vi "_tools_protoc.vi"   [LabVIEW 2020]
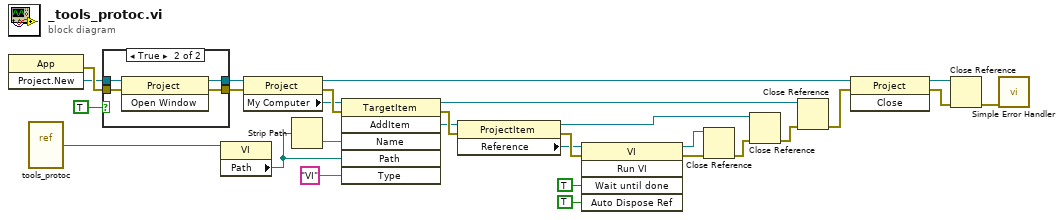
[diagram p0: block diagram]
diagram:
  n1 = invoke class="App" method="Project.New"() -> (error out=w28:errorcluster, "Project:New"=w4:refnum<vi>)  [unwired: 3 in, 1 out]
  n2 = vi-ref "tools_protoc.vi"() -> (w23:refnum<vi>)
  n3 = case shown="True" TRUE {
    tunnel: w4 -> [w30 w34]
    tunnel: w28 -> [w29 w33]
    tunnel: [w30 w32] -> w3
    tunnel: [w29 w31] -> w2
    frame False {
    }
    frame True {
      n4 = invoke class="Project" method="Open Window"(reference=w34, error in=w33) -> (reference out=w32:refnum<vi>, error out=w31:errorcluster)  [unwired: 1 in, 1 out]
    }
  }
  n5 = property class="VI"(reference=w23) -> ("Path"=w22:path)  [unwired: 1 in, 2 out]
  n6 = property class="Project"(reference=w3, error in=w2) -> (reference out=w9:refnum<vi>, error out=w27:errorcluster, "My Computer"=w24:refnum<vi>)
  n7 = Strip Path(path=w22) -> (name=w21:string)  [unwired: 1 out]
  n8 = invoke class="TargetItem" method="AddItem"(reference=w24, error in=w27, "Name"=w21, "Path"=w22, "Type"="VI") -> (reference out=w11:refnum<vi>, error out=w26:errorcluster, "AddItem"=w19:refnum<vi>)  [unwired: 1 in, 3 out]
  n9 = property class="ProjectItem"(reference=w19, error in=w26) -> (reference out=w12:refnum<vi>, error out=w25:errorcluster, "Reference"=w18:refnum<vi>)
  n10 = invoke class="VI" method="Run VI"(reference=w18, error in=w25, "Wait until done"=TRUE ("Wait Until Done"), "Auto Dispose Ref"=TRUE ("Auto Dispose Reference")) -> (reference out=w14:refnum<vi>, error out=w15:errorcluster)  [unwired: 1 in, 3 out]
  n11 = Close Reference(reference=w14, error in (no error)=w15) -> (error out=w13:errorcluster)
  n12 = Close Reference(reference=w12, error in (no error)=w13) -> (error out=w10:errorcluster)
  n13 = Close Reference(reference=w11, error in (no error)=w10) -> (error out=w8:errorcluster)
  n14 = invoke class="Project" method="Close"(reference=w9, error in=w8) -> (reference out=w7:refnum<vi>, error out=w6:errorcluster)  [unwired: 1 in, 1 out]
  n15 = Close Reference(reference=w7, error in (no error)=w6) -> (error out=w5:errorcluster)
  n16 = call <vilib>:"Simple Error Handler.vi"("error in (no error)"=w5) -> ()  [unwired: 4 in, 5 out]
